vi "quadrant-photodiode-subvi.vi"() -> ()   [LabVIEW 2014]
uses:
  tirf-lock-globals.vi
panel:
  in  "sample mode":i32(ring)=10178 items=["Finite Samples"=10178, "Continuous Samples"=10123, "Hardware Timed Single Point"=12522]
  in  "number of readings\n to average":i32=1
  in  "Mode":enum16{"Start", "Read", "End"}(ring)
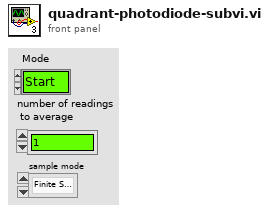
[diagram p1: front panel]
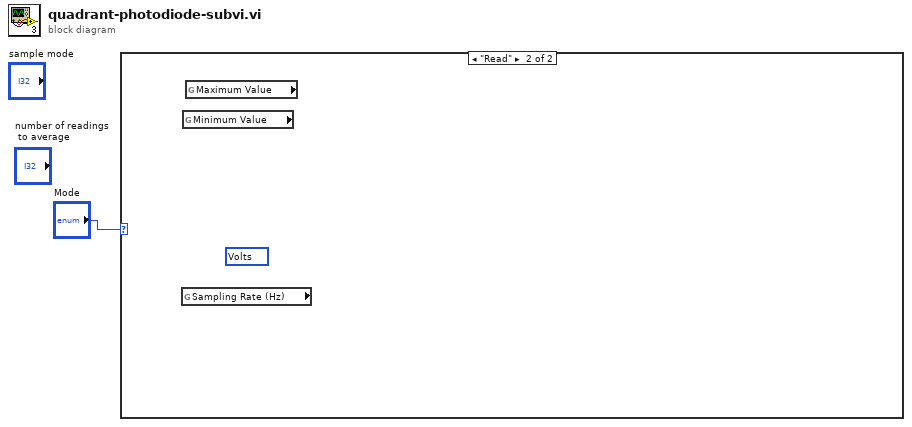
[diagram p0: block diagram]
diagram:
  n1 = case shown="\"Read\"" "Mode" {
    frame "Start", Default {
    }
    frame "Read" {
      (unwired) 10348 items=["Volts"=10348, "From Custom Scale"=10065] ("units")
      n2 = global read "tirf-lock-globals.vi" "Sampling Rate (Hz)"() -> ()  [unwired: 1 out]
      n3 = global read "tirf-lock-globals.vi" "Minimum Value"() -> ()  [unwired: 1 out]
      n4 = global read "tirf-lock-globals.vi" "Maximum Value"() -> ()  [unwired: 1 out]
    }
  }
